vi "test -- fitter -- V2.vi"(1 "MFLI controller action":T4=enum."Scan frequency") -> ()   [LabVIEW 2017]
uses:
  MFLI controller action.ctl
  cursor winow.ctl
  <vilib>/event_ctls.llb/eventvkey.ctl
  peak -- parameters -- complex fit.ctl
  wavepacket.ctl
  filter method control.ctl
  lorentzian.ctl
  circle corners.ctl
  cursor window action.ctl
  plot refs -- filter related.ctl
  publisher action.ctl
  filter - complex - four.vi
  linear interp iiii- complex - z-omega.vi
  peak -- PM find lorenzian - V3.vi
  tale of three indices.vi
  Q -- check range -- i -- real.vi
  filter -- window span logic.vi
  linear interp iiii- complex - z-omega - divide.vi
  linear interpolation iiii- complex.vi
  containing bix.vi
  <vilib>/Analysis/baseanly.llb/A x B.vi
  <vilib>/Analysis/baseanly.llb/Complex A x B.vi
  line -- complex.vi
  Q -- check range -- i -- integer.vi
  peak -- guess at omega -- dzdomega V2.vi
  command stack.vi
  tale of three indices -- check state.vi
  Q - not nan -- real.vi
  Q - not nan -- integer.vi
  peak -- z center from mult phase points.vi
  peak -- estimate for lorentzian.vi
  peak -- fake phase around center.vi
  peak -- get weights.vi
  peak -- four corner circle transformation logic.vi
  peak - fit phase around center - V2.vi
  array - generate range.vi
  circle center from three points.vi
  <vilib>/Utility/error.llb/Clear Errors.vi
  peak -- fit function -- minus arctan.vi
  <vilib>/Analysis/Matrix/Numeric/Conversions/Array To Matrix.vi
  <vilib>/Analysis/Matrix/Numeric/Conversions/Array To Matrix - RA2.vi
  <vilib>/Analysis/baseanly.llb/Inverse Matrix.vi
  <vilib>/Analysis/baseanly.llb/Real Inverse Matrix.vi
  <vilib>/gmath/NumericalOptimization/Nonlinear Curve Fit.vi
  <vilib>/gmath/NumericalOptimization/Nonlinear Curve Fit LM.vi
  KM_filter pipe - plot staff - more - V3.vi
panel:
  in  "Tab :  Fit controls":enum32{"complex plane", "complex plane 2"}(tab)
  in  "Plot: fragment - filter":cluster{dbl[], dbl[]}[](graph)=[{[], []}, {[], []}, {[], []}, {[], []}]
  in  "scale gauge: Plot: complex plane - filter":dbl(slide)=0.00015000000000000001 min=0.0 max=0.3 step=1e-05 scale=0.0001..0.3 scale format="%#_5g"
  in  "Plot: complex plane - filter":cluster{dbl[], dbl[]}[](graph)=[{[], []}, {[], []}, {[0.0, 0.0, 0.0, 0.0, 0.0, 0.0, 0.0, 0.0, 0.0, 0.0, 0.0, 0.0, 0.0, 0.0, 0.0, 0.0, 0.0, 0.0, 0.0, 0.0, 0.0, 0.0, 0.0, 0.0, 0.0, 0.0, 0.0, 0.0, 0.0, 0.0, 0.0, 0.0, 0.0, 0.0, 0.0, 0.0, 0.0, 0.0, 0.0, 0.0, 0.0, 0.0, 0.0, 0.0, 0.0, 0.0, 0.0, 0.0, 0.0, 0.0, 0.0, 0.0, 0.0, 0.0, 0.0, 0.0, 0.0, 0.0, 0.0, 0.0, 0.0, 0.0, 0.0, 0.0, 0.0, 0.0, 0.0, 0.0, 0.0, 0.0, 0.0, 0.0, 0.0, 0.0, 0.0, 0.0, 0.0, 0.0, 0.0, 0.0, 0.0, 0.0, 0.0, 0.0, 0.0, 0.0, 0.0, 0.0, 0.0, 0.0, 0.0, 0.0, 0.0, 0.0, 0.0, 0.0, 0.0, 0.0, 0.0, 0.0], [0.0, 0.0, 0.0, 0.0, 0.0, 0.0, 0.0, 0.0, 0.0, 0.0, 0.0, 0.0, 0.0, 0.0, 0.0, 0.0, 0.0, 0.0, 0.0, 0.0, 0.0, 0.0, 0.0, 0.0, 0.0, 0.0, 0.0, 0.0, 0.0, 0.0, 0.0, 0.0, 0.0, 0.0, 0.0, 0.0, 0.0, 0.0, 0.0, 0.0, 0.0, 0.0, 0.0, 0.0, 0.0, 0.0, 0.0, 0.0, 0.0, 0.0, 0.0, 0.0, 0.0, 0.0, 0.0, 0.0, 0.0, 0.0, 0.0, 0.0, 0.0, 0.0, 0.0, 0.0, 0.0, 0.0, 0.0, 0.0, 0.0, 0.0, 0.0, 0.0, 0.0, 0.0, 0.0, 0.0, 0.0, 0.0, 0.0, 0.0, 0.0, 0.0, 0.0, 0.0, 0.0, 0.0, 0.0, 0.0, 0.0, 0.0, 0.0, 0.0, 0.0, 0.0, 0.0, 0.0, 0.0, 0.0, 0.0, 0.0]}, {[0.0, 0.0, 0.0], [0.0, 0.0, 0.0]}, {[nan, nan, nan, nan, nan, nan, nan, nan, nan, nan, nan, nan, nan, nan, nan, nan, nan, nan, nan, nan], [nan, nan, nan, nan, nan, nan, nan, nan, nan, nan, nan, nan, nan, nan, nan, nan, nan, nan, nan, nan]}, {[0.0, 0.0, 0.0, 0.0, 0.0, 0.0, 0.0, 0.0, 0.0, 0.0, 0.0, 0.0, 0.0, 0.0, 0.0, 0.0, 0.0, 0.0, 0.0, 0.0], [0.0, 0.0, 0.0, 0.0, 0.0, 0.0, 0.0, 0.0, 0.0, 0.0, 0.0, 0.0, 0.0, 0.0, 0.0, 0.0, 0.0, 0.0, 0.0, 0.0]}]
  out "Plot: dz/domega":cluster{"omega out":dbl[], dbl[]}(graph)
  out "Plot: win omega":T1(graph)
  out "Plot: phase":cluster{"omega out":dbl[], dbl[]}(graph)
  out "Plot: phase around center":cluster{dbl[], dbl[]}[](graph)
  out "Plot: fragment":cluster{dbl[], dbl[]}[](graph)
  out "Plot: complex plane":cluster{dbl[], dbl[]}[](graph)=[{[], []}, {[nan, nan, nan, nan, nan, nan, nan, nan, nan, nan, nan, nan, nan, nan, nan, nan, nan, nan, nan, nan, nan, nan, nan, nan, nan, nan, nan, nan, nan, nan, nan, nan, nan, nan, nan, nan, nan, nan, nan, nan, nan, nan, nan, nan, nan, nan, nan, nan, nan, nan], [nan, nan, nan, nan, nan, nan, nan, nan, nan, nan, nan, nan, nan, nan, nan, nan, nan, nan, nan, nan, nan, nan, nan, nan, nan, nan, nan, nan, nan, nan, nan, nan, nan, nan, nan, nan, nan, nan, nan, nan, nan, nan, nan, nan, nan, nan, nan, nan, nan, nan]}, {[nan, nan, nan, nan, nan, nan, nan, nan, nan, nan, nan, nan, nan, nan, nan, nan, nan, nan, nan, nan], [nan, nan, nan, nan, nan, nan, nan, nan, nan, nan, nan, nan, nan, nan, nan, nan, nan, nan, nan, nan]}, {[nan, nan, nan, nan, nan, nan, nan, nan, nan, nan, nan, nan, nan, nan, nan, nan, nan, nan, nan, nan], [nan, nan, nan, nan, nan, nan, nan, nan, nan, nan, nan, nan, nan, nan, nan, nan, nan, nan, nan, nan]}, {[nan, nan, nan, nan, nan, nan, nan, nan, nan, nan, nan, nan, nan, nan, nan, nan, nan, nan, nan, nan], [nan, nan, nan, nan, nan, nan, nan, nan, nan, nan, nan, nan, nan, nan, nan, nan, nan, nan, nan, nan]}, {[nan, nan, nan, nan, nan, nan, nan, nan, nan, nan, nan, nan, nan, nan, nan, nan, nan, nan, nan, nan], [nan, nan, nan, nan, nan, nan, nan, nan, nan, nan, nan, nan, nan, nan, nan, nan, nan, nan, nan, nan]}, {[], []}]
  in  "scale gauge: Plot: complex plane":dbl(slide)=0.00025 min=0.0 max=0.3 step=1e-05 scale=0.0001..1.0 scale format="%#_2g"
  out "pm lorentzian":T2={"Amplitude"=-1.0311345636926572, "omega(0)"=-1.0311345636926572, "Gamma"=-1.0311345636926572, "phase"=-1.0311345636926572, "Q"=-1.0311345636926572, "Norm  Ampl"=-1.0311345636926572, "z (inf)"=-1.0311345636926572+0.0i, "4corners"={"z (-pi/2)"=-1.0311345636926572+0.5736824521422934i, "z(inf)"=-0.5200164984937075+1.0975277942502903i, "z (pi/2)"=-1.0311345636926572+0.5736824521422934i, "z center"=-0.5136528600391839+0.580046090596817i, "z(0)"=-0.5200164984937075+1.0975277942502903i, "radius"=-1.0311345636926572}} {"z (inf)" format="%#9_9f"; "Q" format="%#9_9f"; "phase" format="%#9_9f"; "Gamma" format="%#9_9f"; "omega(0)" format="%#9_9f"}
  in  "plot staff":enum16{"plot", "do not plot", "a"}(ring)
  in  "use fast fit?":bool
  in  "fit?":bool=TRUE
  out "circle gamma (Hz)":dbl format="%#11_11f"
  out "circle phase (rad)":dbl=nan format="%#11_11f"
  out "circle Q":dbl=nan format="%#11_11f"
  out "circle frequency (Hz)":dbl format="%#11_11f"
  in  "all 3":enum32{"all", "other", "other 2"}(tab)
  in  "delay (sec)":dbl=3.0 format="%.3f"
  out "Plot: complex plane - filter":cluster{dbl[], dbl[]}[](graph)
  in  "Stop!":bool
  out "# of points in window":dbl=953.475933538175
  out "window width (kHz)":dbl=76.27809365793496
  out "window center (kHz)":dbl=3399.029286744401
  in  "parameters: complex fit":T5={"main VI path"=path "", "scale factor"=3.0, "# of grid points"=200, "parameters: wavepacket"={"R"=0.5, "wave number"=22.0, "delta k"=7.0, "radii vector"=[], "radial section"=[], "wave vector"=22.0, "wavepacket is"=TRUE}, "span"=0.27789, "interference ?"=enum."cp z center", "filter method"=enum."three"} {"span" min=0.0 max=0.5 step=1e-05 scale=0.0001..0.5 scale format="%#_5f"; "parameters: wavepacket"."delta k" format="%#_3f"; "parameters: wavepacket"."wave number" format="%#_3f"; "parameters: wavepacket"."R" format="%#_3f"}
  out "VKey":T8=enum."Cmd"
  out "Char":i16
  in  "cursor bracket: fit boundaries":T9={"left"=711.3134475992097, "right "=1696.760289361339, "center"=1204.0368684802743, "window"=985.4468417621292, "cursors"=[0, 1, 2], "relative"=2, "absolute"=2, "fixed vertical offset"=0.0, "vertical offset"=0.0, "skew"=0.0, "default window frac"=0.1, "kind"=enum."symmetric", "skew.left"=0.5, "skew.right"=0.5, "Plot ref"=refnum, "wing order"=enum."forw"}
  in  "all":enum32{"all", "other"}(tab)
  out "Plot: hist":cluster{"all rows":dbl[], "all rows":dbl[]}[](graph)
  out "center freq (Hz)":dbl=-0.35260838541595674
  out "window  (Hz)":dbl=17.234446484426172
  out "left freq (Hz)":dbl=-8.969831627629043
  out "right freq (Hz)":dbl=8.26461485679713
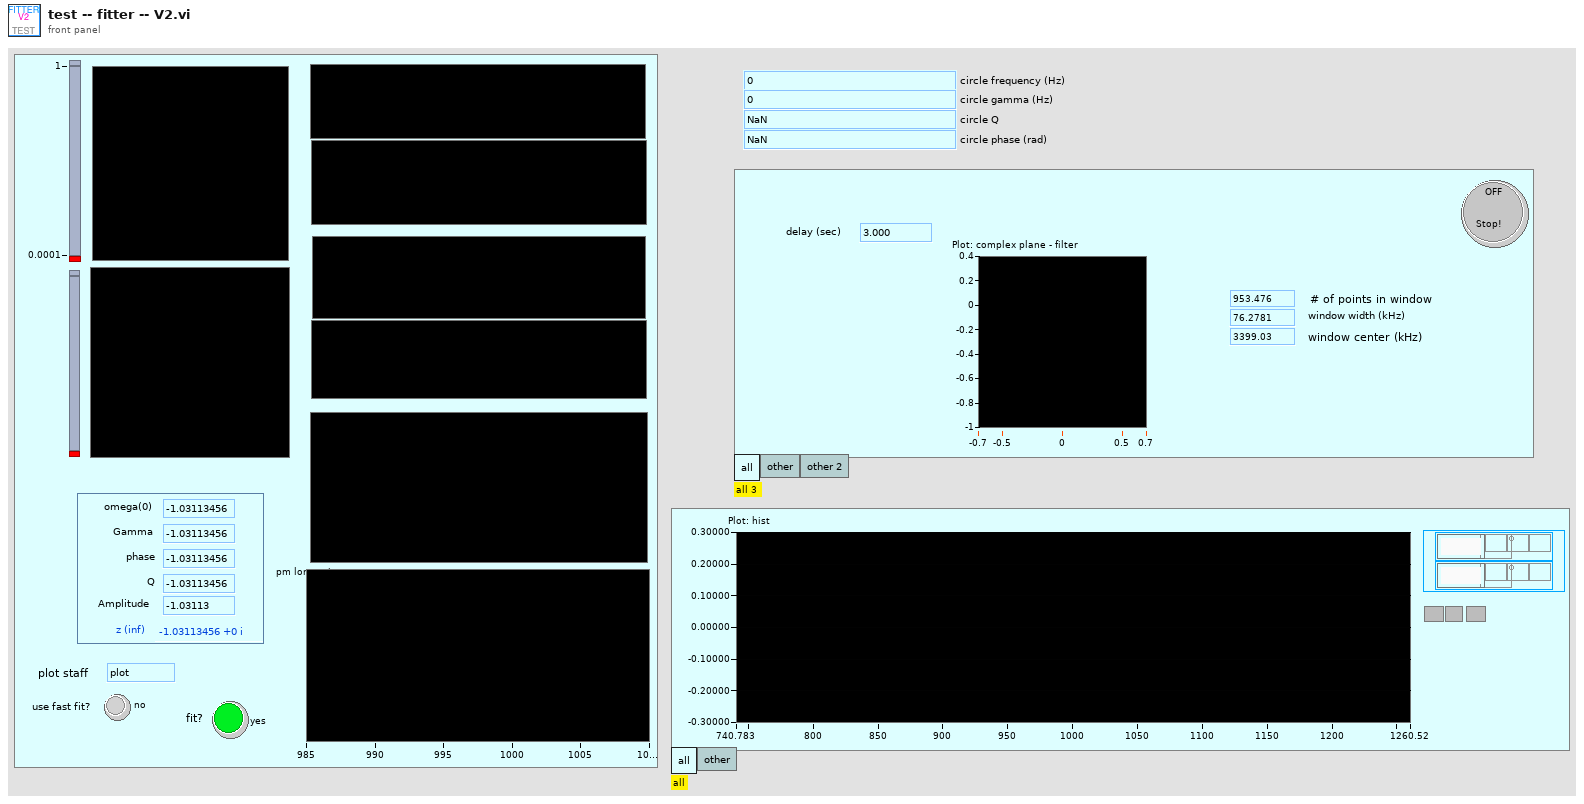
[diagram p1: front panel]
types:
  T1 = cluster{"omega out":dbl[], "win omega out":dbl[]}
  T2 = typedef "lorentzian.ctl" = cluster{"Amplitude":dbl, "omega(0)":dbl, "Gamma":dbl, "phase":dbl, "Q":dbl, "Norm  Ampl":dbl, "z (inf)":cdb, "4corners":T3}
  T3 = typedef "circle corners.ctl" = cluster{"z (-pi/2)":cdb, "z(inf)":cdb, "z (pi/2)":cdb, "z center":cdb, "z(0)":cdb, "radius":dbl}
  T4 = typedef "MFLI controller action.ctl" = enum16{"Initialize", "Scan frequency", "open", "close", "read", "circle PLL"}
  T5 = typedef "peak -- parameters -- complex fit.ctl" = cluster{"main VI path":path, "scale factor":dbl, "# of grid points":i32, "parameters: wavepacket":T6, "span":dbl, "interference ?":enum16{"cp z center", "pm zcenter", "fancy"}, "filter method":T7}
  T6 = typedef "wavepacket.ctl" = cluster{"R":dbl, "wave number":dbl, "delta k":dbl, "radii vector":dbl[], "radial section":cdb[], "wave vector":dbl, "wavepacket is":bool}
  T7 = typedef "filter method control.ctl" = enum16{"four", "five", "one", "two", "three", "zero", "minus one", "minus two"}
  T8 = typedef "eventvkey.ctl" = enum16{"ASCII", "Enter", "Return", "Shift", "Ctrl", "Alt", "Cmd", "Opt", "Caps", "NumLock", "Clear", "Break", "Up", "Down", "Left", "Right", "Insert", "Delete", "Home", "End", "PageUp", "PageDown", "Escape", "Help", "Pause", "ScrollLock", "F1", "F2", "F3", "F4", "F5", "F6", "F7", "F8", "F9", "F10", "F11", "F12", "F13", "F14", "F15", "F16", "F17", "F18", "F19", "F20", "F21", "F22", "F23", "F24", "Play", "VolumeUp", "VolumeDown", "Mute", "Two Byte Char"}
  T9 = typedef "cursor winow.ctl" = cluster{"left":dbl, "right ":dbl, "center":dbl, "window":dbl, "cursors":i32[], "relative":i32, "absolute":i32, "fixed vertical offset":dbl, "vertical offset":dbl, "skew":dbl, "default window frac":dbl, "kind":enum16{"symmetric", "skewed", "fancy"}, "skew.left":dbl, "skew.right":dbl, "Plot ref":refnum<vi>, "wing order":enum16{"forw", "back"}}
  T10 = typedef "plot refs -- filter related.ctl" = cluster{"Plot: complex plane - filter":refnum<vi>, "Plot: dz/domega":refnum<vi>, "Plot: fragment filter":refnum<vi>, "Plot: win omega":refnum<vi>, "Plot: phase":refnum<vi>, "Plot: phase around center":refnum<vi>, "Plot: complex plane":refnum<vi>, "Plot: fragment":refnum<vi>}
  T11 = typedef "cursor window action.ctl" = enum16{"balance", "h. offset change", "cursor moves", "change center", "change window", "init", "check", "reset", "set y to middle", "idle", "-write all Y", "-write left.X", "-write center.X", "-write right.X", "-write all X", "-change center", "-change window", "-change skew", "-read cursor 2", "-read cursor 1", "-read cursor 0", "-read all cursors", "-reset", "-read plot scale", "-set y to middle", "-Q: center.Y is visible", "-Q: window is visible", "-parse center.Y", "-right left from center", "-left move", "-right move", "-set center.Y", "-empty", "-set cursors to default", "-check", "-write center.Y", "-copy cursor 1", "-copy cursor 0", "-copy cursor 2", "move right", "move left", "shrink", "broaden", "skew up", "skew down", "-write plot scale", "zoom X", "change cen&win", "zoom to all data", "color--red", "color--green", "color--yellow", "read", "zoom out", "zoom in", "slide right", "slide left"}
  T12 = typedef "publisher action.ctl" = enum16{"set", "get"}
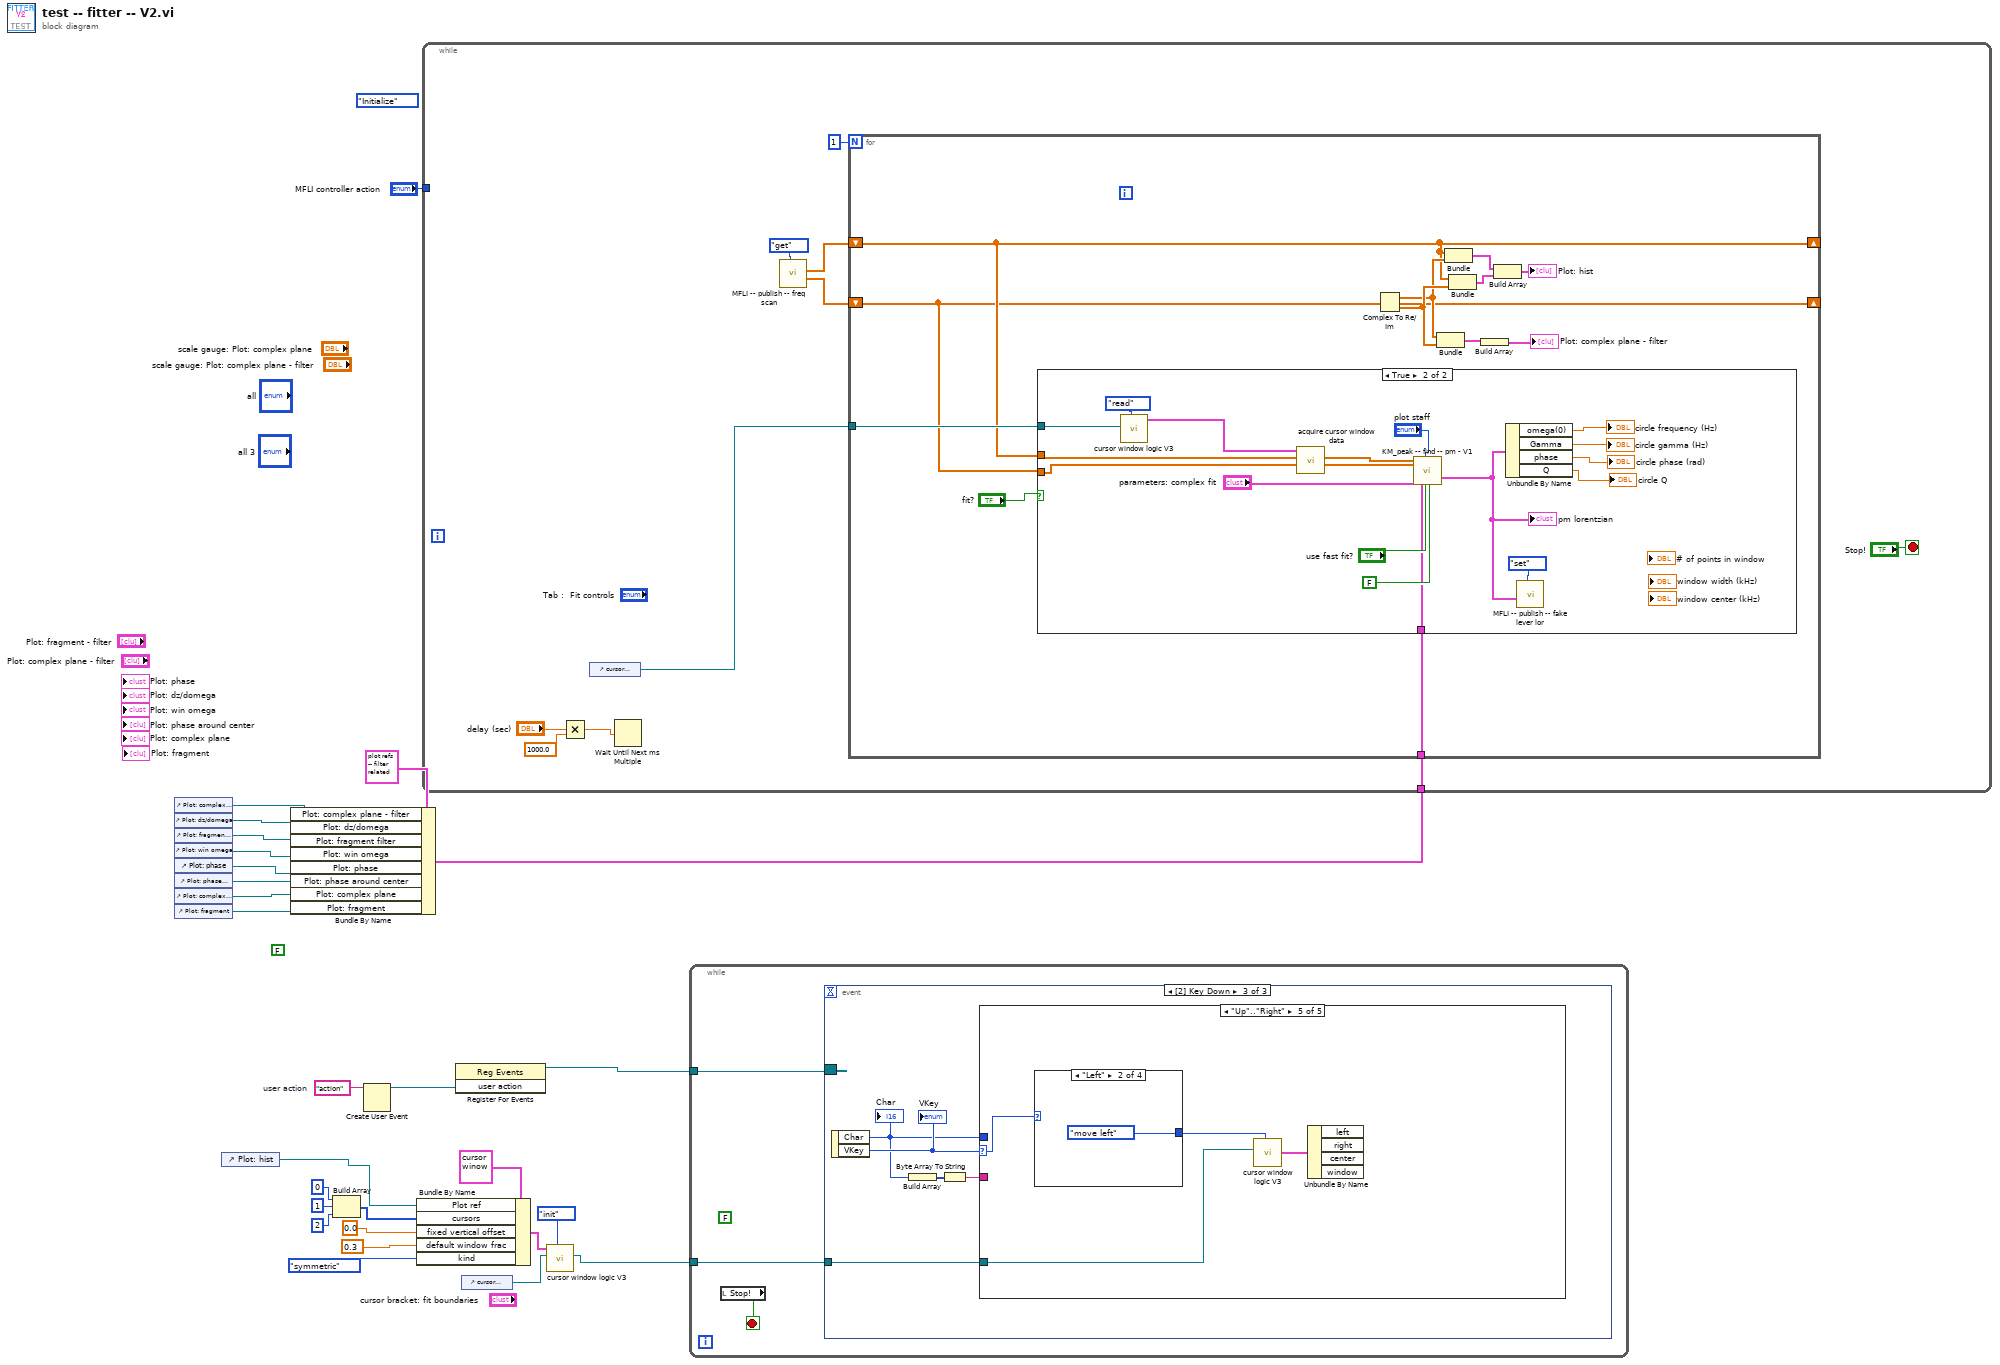
[diagram p0: block diagram]
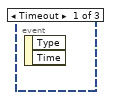
[diagram p2: hidden frame]
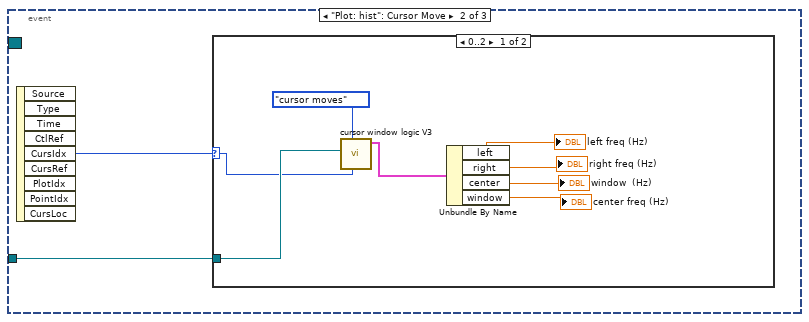
[diagram p3: hidden frame]
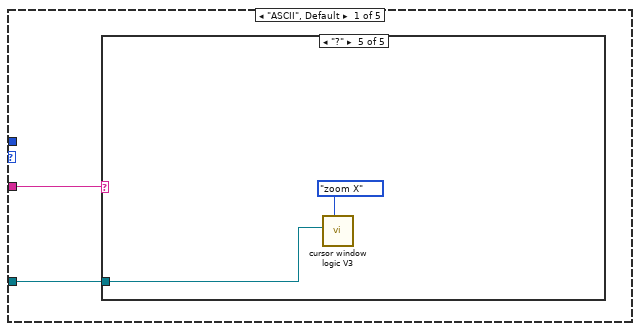
[diagram p5: hidden frame]
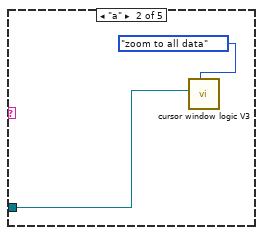
[diagram p7: hidden frame]
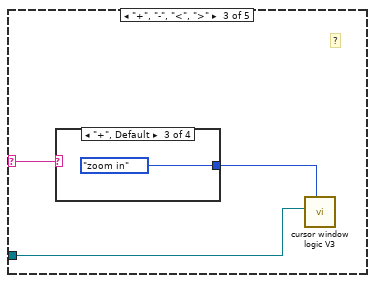
[diagram p8: hidden frame]
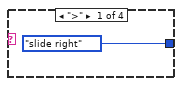
[diagram p9: hidden frame]
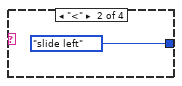
[diagram p10: hidden frame]
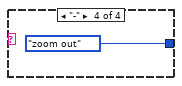
[diagram p11: hidden frame]
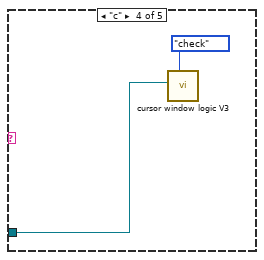
[diagram p12: hidden frame]
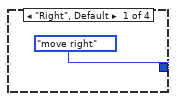
[diagram p16: hidden frame]
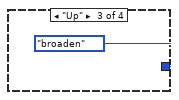
[diagram p17: hidden frame]
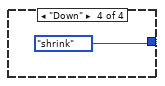
[diagram p18: hidden frame]
diagram:
  (unwired) FALSE
  w24 = "action"  # user action
  (unwired) MFLI_controller_action."Initialize" ("MFLI controller action")
  n1 = control-ref of="Plot: complex plane - filter"() -> (w10:refnum<vi>)
  n2 = control-ref of="Plot: dz/domega"() -> (w9:refnum<vi>)
  n3 = control-ref of="Plot: fragment - filter"() -> (w8:refnum<vi>)
  n4 = control-ref of="Plot: win omega"() -> (w7:refnum<vi>)
  n5 = control-ref of="Plot: phase"() -> (w6:refnum<vi>)
  n6 = control-ref of="Plot: phase around center"() -> (w5:refnum<vi>)
  n7 = control-ref of="Plot: complex plane"() -> (w4:refnum<vi>)
  n8 = control-ref of="Plot: fragment"() -> (w3:refnum<vi>)
  n9 = control-ref of="Plot: hist"() -> (w11:refnum<vi>)
  n10 = Bundle By Name(cluster=T10 {"Plot: complex plane - filter"=refnum, "Plot: dz/domega"=refnum, "Plot: fragment filter"=refnum, "Plot: win omega"=refnum, "Plot: phase"=refnum, "Plot: phase around center"=refnum, "Plot: complex plane"=refnum, "Plot: fragment"=refnum} ("plots: filter related"), "Plot: complex plane - filter"=w10, "Plot: dz/domega"=w9, "Plot: fragment filter"=w8, "Plot: win omega"=w7, "Plot: phase"=w6, "Plot: phase around center"=w5, "Plot: complex plane"=w4, "Plot: fragment"=w3) -> (w2:T10)
  n11 = Build Array(0, 1, 2) -> (w12:i32[])
  n12 = Create User Event(user event datatype=w24) -> (user event=w25:refnum<user-event>)  [unwired: 1 in, 1 out]
  n13 = Bundle By Name(cluster=T9 {"left"=0.0, "right "=0.0, "center"=0.0, "window"=0.0, "cursors"=[], "relative"=0, "absolute"=0, "fixed vertical offset"=0.0, "vertical offset"=0.0, "skew"=0.0, "default window frac"=0.0, "kind"=enum."symmetric", "skew.left"=0.0, "skew.right"=0.0, "Plot ref"=refnum, "wing order"=enum."forw"} ("cursor bracket: All, data window"), "Plot ref"=w11, "cursors"=w12, "fixed vertical offset"=0.0, "default window frac"=0.3 ("fixed vertical offset"), "kind"=enum16{"symmetric", "skewed", "fancy"}."symmetric") -> (w20:T9)
  n14 = while {
    tunnel: "MFLI controller action" -> [_]
    tunnel: w2 -> [w32]
    stop <- "Stop!" stop-if-true
    n15 = Multiply(x="delay (sec)", y=1000.0) -> (x*y=w28:dbl)
    n16 = control-ref of="cursor bracket: fit boundaries"() -> (w33:refnum<vi>)
    n17 = Wait Until Next ms Multiple(millisecond multiple=w28) -> ()  [unwired: 1 out]
    n18 = call "MFLI -- publish -- freq scan.vi"("publisher action"=publisher_action."get") -> ("Voltage out (V)"=w34:cdb[], "Freq out (Hz)"=w35:dbl[])  [unwired: 9 in]
    n19 = for {
      N: 1 -> [_]
      shift-right: [w40] -> _
      shift-left: w34 -> [w40]
      shift-right: [w41] -> _
      shift-left: w35 -> [w41]
      tunnel: w33 -> [w42]
      tunnel: w32 -> [w38]
      n20 = case shown="True" "fit?" {
        tunnel: w42 -> [_ w62]
        tunnel: w41 -> [_ w60]
        tunnel: w40 -> [_ w57]
        tunnel: w38 -> [_ w52]
        frame False {
        }
        frame True {
          n21 = call "cursor window logic V3.vi"("cursor window action"=cursor_window_action."read", "cursor window in"=w62) -> ("cursor window out"=w58:T9)  [unwired: 8 in, 1 out]
          n22 = call "acquire cursor window data.vi"("z in"=w57, "omega in"=w60, "cursor window"=w58) -> ("z out"=w59:cdb[], "omega  out"=w61:dbl[])  [unwired: 4 in, 3 out]
          n23 = call "KM_peak -- find -- pm - V1.vi"("omega in"=w61, "z in"=w59, "parameters: complex fit"="parameters: complex fit", "plots: filter related"=w52, "plot staff ?"="plot staff", "just guess?"="use fast fit?", "subtract linear BG"=FALSE) -> ("pm lorentzian"=w50:T2)  [unwired: 10 in, 2 out]
          "pm lorentzian" <- w50
          n24 = Unbundle By Name(w50) -> ("omega(0)"=→"circle frequency (Hz)":dbl, "Gamma"=→"circle gamma (Hz)":dbl, "phase"=→"circle phase (rad)":dbl, "Q"=→"circle Q":dbl)
          n25 = call "MFLI -- publish -- fake lever lor.vi"("publisher action"=publisher_action."set", "lorentzian IN"=w50) -> ()  [unwired: 9 in, 1 out]
        }
      }
      n26 = Complex To Re/Im(x + iy=w40) -> (x=w45:dbl[], y=w46:dbl[])
      n27 = Bundle(w45, w46) -> (w39:cluster{dbl[], dbl[]})  [unwired: 1 in]
      n28 = Bundle("Freq out (Hz)"=w41, w45) -> (w49:cluster{"Freq out (Hz)":dbl[], dbl[]})  [unwired: 1 in]
      n29 = Bundle("Freq out (Hz)"=w41, w46) -> (w48:cluster{"Freq out (Hz)":dbl[], dbl[]})  [unwired: 1 in]
      n30 = Build Array(w39) -> (→"Plot: complex plane - filter":cluster{dbl[], dbl[]}[])
      n31 = Build Array(w49, w48) -> (→"Plot: hist":cluster{"Freq out (Hz)":dbl[], dbl[]}[])
    }
  }
  n32 = register-events(w25) -> (reference out=w23:refnum<event-registration>)  [unwired: 2 in, 1 out]
  n33 = control-ref of="cursor bracket: fit boundaries"() -> (w22:refnum<vi>)
  n34 = call "cursor window logic V3.vi"("cursor window action"=cursor_window_action."init", "cursor window in"=w22, "cursor window init"=w20) -> ("cursor window out"=w26:refnum<vi>)  [unwired: 7 in, 1 out]
  n35 = while {
    tunnel: w23 -> [w70]
    tunnel: w26 -> [w69]
    stop <- w68 stop-if-true
    (unwired) FALSE
    n36 = local read "Stop!"() -> (w68:bool)
    n37 = event shown="[2] Key Down" {
      selector: w70 -> [_ _ _]
      dyn-events: _ -> [_ _ _]
      timeout: _ -> [_ _ _]
      tunnel: w69 -> [_ w72 w81]
      event Timeout {
        n38 = event-data() -> ()  [unwired: 1 in, 2 out]
      }
      event "Plot: hist": Cursor Move {
        n39 = event-data() -> ("CursIdx"=w71:i32)  [unwired: 1 in, 8 out]
        n40 = case shown="0..2" w71 {
          selector: w71 -> [w78 _]
          tunnel: w72 -> [w80 _]
          frame 0..2 {
            n41 = call "cursor window logic V3.vi"("CursIdx"=w78, "cursor window action"=cursor_window_action."cursor moves", "cursor window in"=w80) -> ("cursor window out"=w77:T9)  [unwired: 7 in, 1 out]
            n42 = Unbundle By Name(w77) -> ("left"=→"left freq (Hz)":dbl, "right"=→"right freq (Hz)":dbl, "center"=→"window  (Hz)":dbl, "window"=→"center freq (Hz)":dbl)
          }
          frame 3, Default {
          }
        }
      }
      event Key Down {
        n43 = event-data() -> ("Char"=w83:i16, "VKey"=w85:T8)  [unwired: 1 in]
        "Char" <- w83
        "VKey" <- w85
        n44 = Build Array(w83) -> (w84:i16[])
        n45 = Byte Array To String(unsigned byte array=w84) -> (string=w82:string)
        n46 = case shown="\"Up\"..\"Right\"" w85 {
          selector: w85 -> [_ _ _ _ w104]
          tunnel: w83 -> [_ _ _ _ _]
          tunnel: w82 -> [w87 _ _ _ _]
          tunnel: w81 -> [w86 _ _ _ w101]
          frame "ASCII", Default {
            n47 = case shown="\"?\"" w87 {
              selector: w87 -> [_ _ w91 _ _]
              tunnel: w86 -> [_ w88 w92 w97 w99]
              frame "0", Default {
              }
              frame "a" {
                n48 = call "cursor window logic V3.vi"("cursor window action"=cursor_window_action."zoom to all data", "cursor window in"=w88) -> ()  [unwired: 8 in, 2 out]
              }
              frame "+", "-", "<", ">" {
                # "?"
                n49 = case shown="\"+\", Default" w91 {
                  tunnel: [cursor_window_action."slide right" ("cursor window action") cursor_window_action."slide left" ("cursor window action") cursor_window_action."zoom in" ("cursor window action") cursor_window_action."zoom out" ("cursor window action")] -> w90
                  frame ">" {
                  }
                  frame "<" {
                  }
                  frame "+", Default {
                  }
                  frame "-" {
                  }
                }
                n50 = call "cursor window logic V3.vi"("cursor window action"=w90, "cursor window in"=w92) -> ()  [unwired: 8 in, 2 out]
              }
              frame "c" {
                n51 = call "cursor window logic V3.vi"("cursor window action"=cursor_window_action."check", "cursor window in"=w97) -> ()  [unwired: 8 in, 2 out]
              }
              frame "?" {
                n52 = call "cursor window logic V3.vi"("cursor window action"=cursor_window_action."zoom X", "cursor window in"=w99) -> ()  [unwired: 8 in, 2 out]
              }
            }
          }
          frame "Escape" {
          }
          frame "PageUp" {
          }
          frame "PageDown" {
          }
          frame "Up".."Right" {
            n53 = case shown="\"Left\"" w104 {
              tunnel: [cursor_window_action."move right" ("cursor window action") cursor_window_action."move left" ("cursor window action") cursor_window_action."broaden" ("cursor window action") cursor_window_action."shrink" ("cursor window action")] -> w103
              frame "Right", Default {
              }
              frame "Left" {
              }
              frame "Up" {
              }
              frame "Down" {
              }
            }
            n54 = call "cursor window logic V3.vi"("cursor window action"=w103, "cursor window in"=w101) -> ("cursor window out"=w102:T9)  [unwired: 8 in, 1 out]
            n55 = Unbundle By Name(w102) -> ()  [unwired: 4 out]
          }
        }
      }
    }
  }
